vi "Stop.vi"(8 "error in (no error)":errorcluster, 11 "Electrophysiology in":refnum<class "BehaviorData.lvclass">) -> (0 "error out":errorcluster, 3 "Electrophysiology out":refnum<class "BehaviorData.lvclass">)   [LabVIEW 2014, in "BehaviorData.lvclass"]
uses:
  BehaviorData.lvclass
  BehaviorData.lvclass/BehaviorData.ctl
  AcquireTraces/AcquireTraces.lvclass
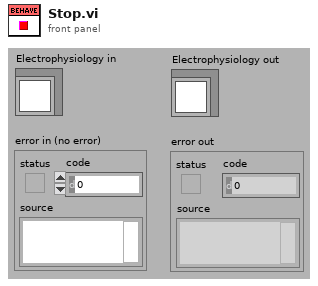
[diagram p1: front panel]
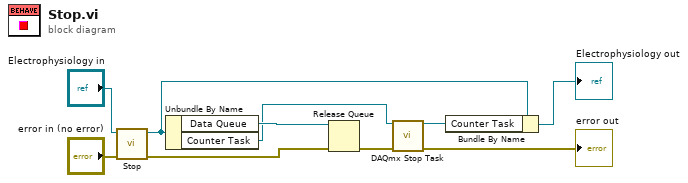
[diagram p0: block diagram]
diagram:
  n1 = call-parent "Stop.vi"("error in (no error)"="error in (no error)", "Electrophysiology in"="Electrophysiology in") -> ("error out"=w5:errorcluster, "Electrophysiology out"=w3:refnum<class "BehaviorData.lvclass">)  [unwired: 8 in]
  n2 = Unbundle By Name(w3) -> ("Data Queue"=w8:refnum<queue>, "Counter Task"=w7:refnum<k21>)
  n3 = Release Queue(queue=w8, error in (no error)=w5) -> (error out=w6:errorcluster)  [unwired: 1 in, 2 out]
  n4 = call <vilib>:"DAQmx Stop Task.vi"("task/channels in"=w7, "error in"=w6) -> ("task out"=w2:refnum<k21>, "error out"=→"error out":errorcluster)  [unwired: 12 in]
  n5 = Bundle By Name(cluster=w3, "Counter Task"=w2) -> (→"Electrophysiology out":refnum<class "BehaviorData.lvclass">)
